vi "Close.vi"(8 "error in (no error)":errorcluster, 11 "PSU_N87 in":refnum<class "PSU_N67.lvclass">) -> (0 "error out":errorcluster)   [LabVIEW 2014, in "PSU_N67.lvclass"]
uses:
  PSU_N67.lvclass
  PSU.lvclass/PSU.ctl
  PSU_N67.lvclass/PSU_N67.ctl
  Read Channel.vi
  <instrlib>/Agilent N6700 Series/Agilent N6700 Series.lvlib
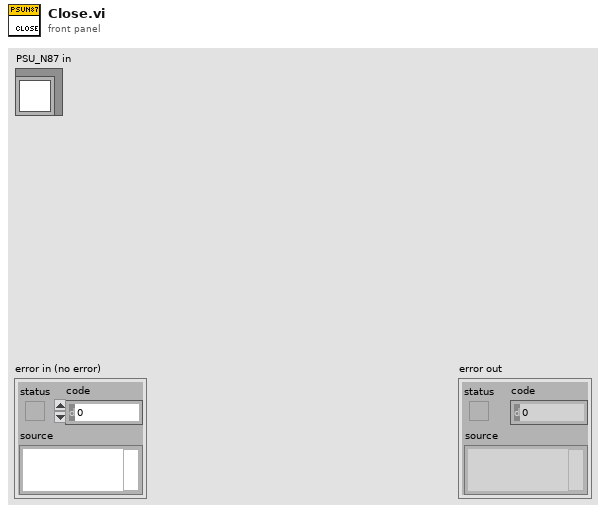
[diagram p1: front panel]
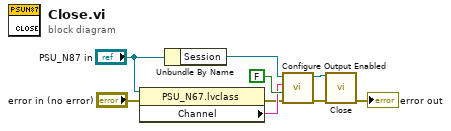
[diagram p0: block diagram]
diagram:
  n1 = property class="PSU_N67.lvclass"(reference="PSU_N87 in", error in="error in (no error)") -> (error out=w1:errorcluster, "Channel"=w3:string)  [unwired: 1 out]
  n2 = Unbundle By Name("PSU_N87 in") -> ("Session"=w5:refnum<visa-resource-name>)
  n3 = call <instrlib>:"Configure Output Enabled.vi"("error in (no error)"=w1, "Enable Output (False)"=FALSE, "Channel Name (1)"=w3, "VISA resource name"=w5) -> ("error out"=w7:errorcluster, "VISA resource name out"=w8:refnum<visa-resource-name>)  [unwired: 6 in]
  n4 = call <instrlib>:"Close.vi"("VISA resource name"=w8, "error in (no error)"=w7) -> ("error out"=→"error out":errorcluster)  [unwired: 13 in]
